vi "Dictionary To CSV.vi"(0 "Dictionary":refnum<class "Dictionary.lvclass">, 11 "Error in":errorcluster caption="Error in (no error)") -> (4 "CSV String":string, 15 "Error out":errorcluster)   [LabVIEW 2018, in "Dictionary - CSV.lvlib"]
doc: "Converting <B>Dictionary</B> to <B>CSV String</B>.\n\nThis VI runs only if there is no error on <B>Error in</B>.\n\nKåre Juul Kirkegaard\nGPower\n5/4 2019"
uses:
  <vilib>/GPower/Dictionary/Library/Dictionary Class/Dictionary.lvclass
  0daabf8c-ee7c-4f17-95c7-9a994888c811.vi
  ece3dd93-42b9-4407-a7f9-9e323b9c5b55.vi
  <vilib>/GPower/Dictionary/Library/Dictionary Class/Get/Get Path.vi
  Dictionary - CSV.lvlib
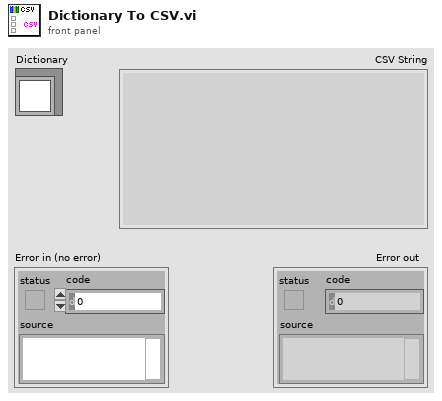
[diagram p1: front panel]
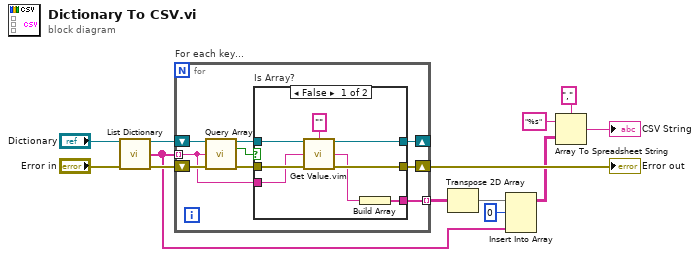
[diagram p0: block diagram]
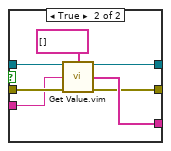
[diagram p2: hidden frame]
diagram:
  n1 = call <vilib>:"List Dictionary.vi"("Dictionary in"="Dictionary", "Error in"="Error in") -> ("Dictionary out"=w12:refnum<class "Dictionary.lvclass">, "Keys"=w6:string[], "Error out"=w11:errorcluster)  [unwired: 11 in]
  n2 = for "For each key..." {
    tunnel: w6 -> [w14] mode=indexing
    shift-right: [w15] -> w7
    shift-left: w11 -> [w21]
    shift-right: [w17] -> _
    shift-left: w12 -> [w22]
    tunnel: [w16] -> w5 mode=indexing
    n3 = call <vilib>:"Query Array.vi"("Dictionary in"=w22, "Key Path"=w14, "Error in"=w21) -> ("Dictionary out"=w18:refnum<class "Dictionary.lvclass">, "Is Array?"=w20:bool, "Error out"=w19:errorcluster)  [unwired: 9 in, 1 out]
    n4 = case "Is Array?" shown="False" w20 {
      tunnel: w19 -> [w28 w37]
      tunnel: w18 -> [w27 w36]
      tunnel: [w30 w34] -> w17
      tunnel: [w24 w33] -> w16
      tunnel: [w29 w32] -> w15
      tunnel: w14 -> [w23 w31]
      frame False {
        n5 = call "Get Value.vim"("Dictionary in"=w27, "Value Type"="", "Key Path"=w23, "Error in"=w28) -> ("Dictionary out"=w30:refnum<class "Dictionary.lvclass">, "Value"=w25:string, "Error out"=w29:errorcluster)  [unwired: 9 in]
        n6 = Build Array(w25) -> (w24:string[])
      }
      frame True {
        n7 = call "Get Value.vim"("Dictionary in"=w36, "Value Type"=string[] [], "Key Path"=w31, "Error in"=w37) -> ("Dictionary out"=w34:refnum<class "Dictionary.lvclass">, "Value"=w33:string[], "Error out"=w32:errorcluster)  [unwired: 9 in]
      }
    }
  }
  "Error out" <- w7
  n8 = Transpose 2D Array(2D array=w5) -> (transposed array=w2:string[][])
  n9 = Insert Into Array(array=w2, index (row)=0, new element=w6) -> (w4:string[][])  [unwired: 1 in]
  n10 = Array To Spreadsheet String(delimiter (Tab)=",", array=w4, 3:"%s" ("format string")) -> (spreadsheet string=→"CSV String":string)
